vi "PID Online Autotuning (Relay Feedback).vi"(0 "setpoint":dbl(slide)=30.8641975308642 scale=0.0..100.0 scale format="%.1f", 1 "manipulated variable":dbl(slide)=30.8641975308642 scale=0.0..100.0 scale format="%.1f", 3 "autotuning parameters":T2={"type of controller"=1, "relay cycles"=3, "relay amplitude"=1.0, "control specifications"=2, "PV noise level"=0.1} {"PV noise level" format="%.2f"; "control specifications" items=["Fast", "Normal", "Slow"]; "relay amplitude" format="%.2f"; "type of controller" items=["P", "PI", "PID"]}, 5 "process variable":dbl(slide)=19.583333333333336 scale=0.0..100.0 scale format="%.1f", 9 "PID gains in":T1={"proportional gain (Kc)"=1.0, "integral time (Ti, min)"=0.01, "derivative time (Td, min)"=0.0} {"derivative time (Td, min)" format="%.3f"; "integral time (Ti, min)" format="%.3f"; "proportional gain (Kc)" format="%.3f"}, 11 "dt (s)":dbl=-1.0 format="%.3f", 12 "reinitialize? (F)":bool, 13 "autotune? (F)":bool) -> (4 "setpoint out":dbl(slide)=30.8641975308642 scale=0.0..100.0 scale format="%.1f", 6 "process variable out":dbl(slide)=19.583333333333336 scale=0.0..100.0 scale format="%.1f", 8 "tuning completed?":bool, 10 "PID gains out":T1={"proportional gain (Kc)"=1.0, "integral time (Ti, min)"=0.01, "derivative time (Td, min)"=0.0} {"derivative time (Td, min)" format="%.3f"; "integral time (Ti, min)" format="%.3f"; "proportional gain (Kc)" format="%.3f"}, 14 "tuned PID gains":T1={"proportional gain (Kc)"=1.0, "integral time (Ti, min)"=0.01, "derivative time (Td, min)"=0.0} {"derivative time (Td, min)" format="%.3f"; "integral time (Ti, min)" format="%.3f"; "proportional gain (Kc)" format="%.3f"})   [LabVIEW 2020, in "NI_PID_autopid.lvlib"]
doc: "Controls the parameters of a PID controller based on the autotuning technique of the polymorphic instance you select. You can use this VI in applications with other PID VIs, such as PID or PID Advanced, to construct and tune a PID controller. You must manually select the polymorphic instance to use."
uses:
  <vilib>/addons/control/pid/NI_PID_autopid.lvlib
  <vilib>/addons/control/pid/autopid.llb/PID autotuning parameters.ctl
  <vilib>/addons/control/pid/pid.llb/PID Structure Conversion (DBL).vi
  <vilib>/addons/control/pid/NI_PID_pid.lvlib
panel:
  in  "relay setpoint":bool
  in  "calculate parameters":bool
  # "Relay PID Auto Tune"
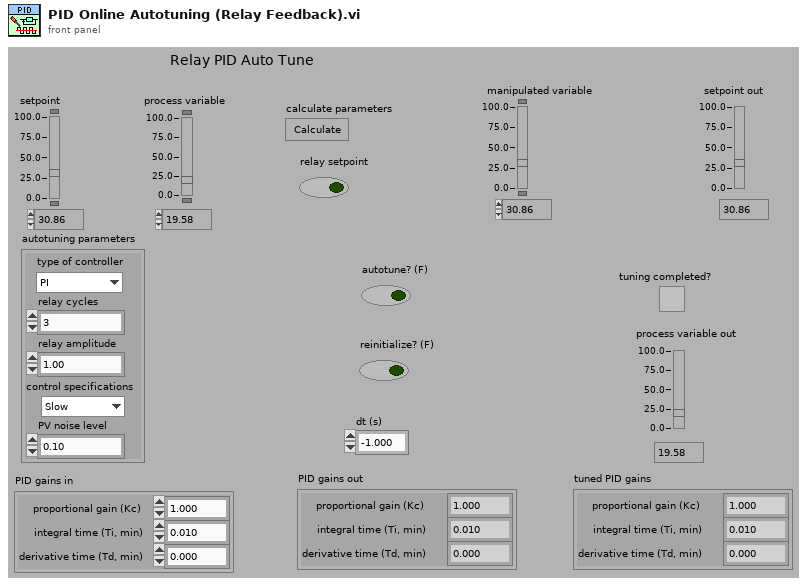
[diagram p1: front panel]
types:
  T1 = cluster{"proportional gain (Kc)":dbl, "integral time (Ti, min)":dbl, "derivative time (Td, min)":dbl}
  T2 = typedef "PID autotuning parameters.ctl" = cluster{"type of controller":u16, "relay cycles":i32, "relay amplitude":dbl, "control specifications":u16, "PV noise level":dbl}
  T3 = enum16{"Academic (Standard)", "Parallel", "Series"}
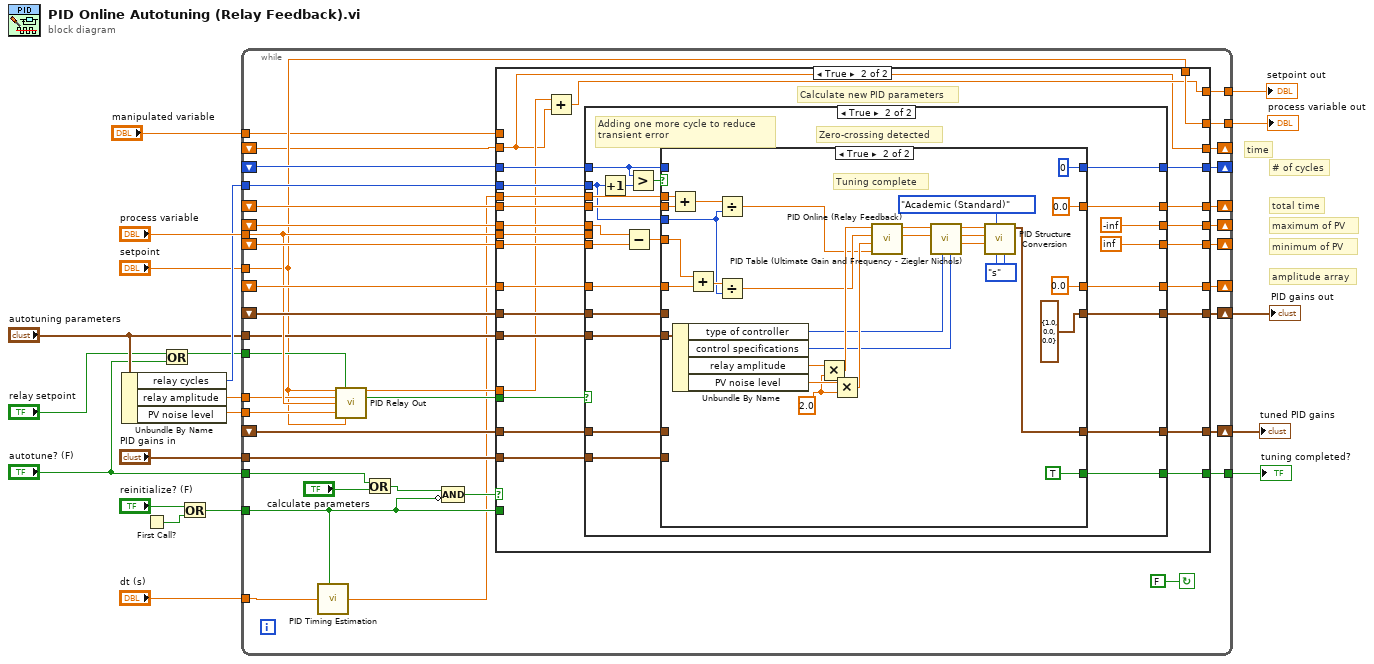
[diagram p0: block diagram]
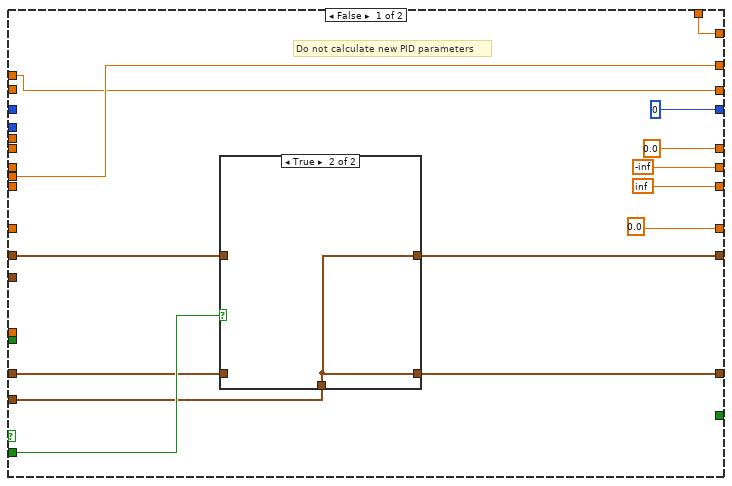
[diagram p2: hidden frame]
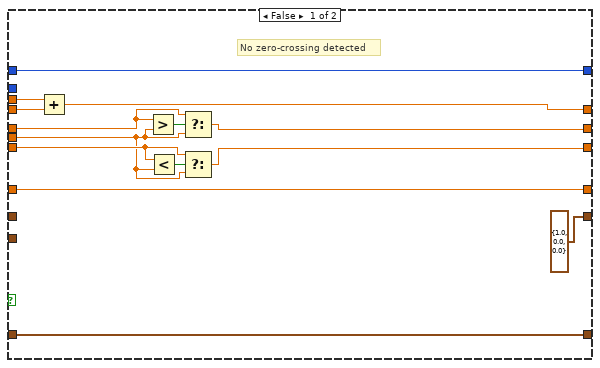
[diagram p4: hidden frame]
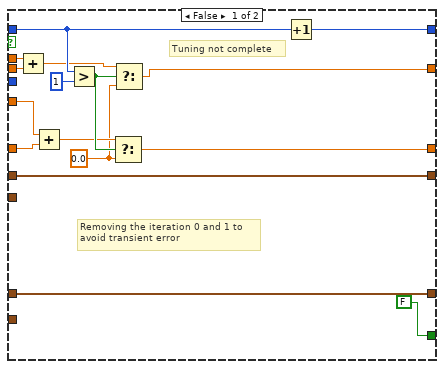
[diagram p5: hidden frame]
diagram:
  # "time"
  # "amplitude array"
  # "total time"
  # "minimum of PV"
  # "maximum of PV"
  # "# of cycles"
  n1 = Unbundle By Name("autotuning parameters") -> ("relay cycles"=w15:i32, "relay amplitude"=w11:dbl, "PV noise level"=w10:dbl)
  n2 = First Call?() -> (First Call?: T/F=w17:bool)
  n3 = Or(x="relay setpoint", y="autotune? (F)") -> (x .or. y?=w7:bool)
  n4 = Or(x="reinitialize? (F)", y=w17) -> (x .or. y?=w9:bool)
  n5 = while {
    shift-left: _ -> [w49]
    shift-right: [w48] -> _
    shift-left: _ -> [w50]
    shift-right: [w46] -> w20
    shift-left: _ -> [w53]
    shift-right: [w54] -> _
    shift-left: _ -> [w52]
    shift-right: [w55] -> _
    shift-left: _ -> [w56]
    shift-right: [w57] -> _
    shift-left: _ -> [w51]
    shift-right: [w58] -> _
    tunnel: w9 -> [w22]
    tunnel: "dt (s)" -> [w23]
    tunnel: "process variable" -> [w43]
    tunnel: w15 -> [w42]
    tunnel: w10 -> [w41]
    tunnel: w11 -> [w40]
    tunnel: "autotuning parameters" -> [w39]
    tunnel: "PID gains in" -> [w38]
    tunnel: "setpoint" -> [w32]
    tunnel: w7 -> [w37]
    tunnel: "autotune? (F)" -> [w34]
    tunnel: [w33] -> w5
    tunnel: [w30] -> w4
    tunnel: "manipulated variable" -> [w29]
    shift-right: [w28] -> _
    shift-left: _ -> [w27]
    tunnel: [w26] -> w2
    shift-right: [w25] -> w1
    shift-left: _ -> [w24]
    stop <- FALSE continue-if-true
    n6 = call <vilib>:"PID Timing Estimation.vi"("Initialize?"=w22, "dt (s) in"=w23) -> ("dt (s) out"=w21:dbl)  [unwired: 7 in]
    n7 = call <vilib>:"PID Relay Out.vi"("Setpoint Reference"=w32, "Relay Setpoint"=w37, "Relay Amplitude"=w40, "Process Variable"=w43, "Noise Disturbance"=w41, "Process Variable Reference"=w32) -> ("relay output"=w31:dbl, "Zero Crossing"=w36:bool)  [unwired: 2 in, 6 out]
    n8 = Or(x=w34, y="calculate parameters") -> (x .or. y?=w35:bool)
    n9 = Compound Arithmetic op=AND(w35, invert w22) -> (w44:bool)
    n10 = case shown="True" w44 {
      tunnel: w51 -> [_ w89]
      tunnel: [0 w90] -> w58
      tunnel: [-inf w91] -> w57
      tunnel: w56 -> [_ w100]
      tunnel: w52 -> [_ w99]
      tunnel: [0.0 w93] -> w55
      tunnel: [inf w92] -> w54
      tunnel: w53 -> [_ w94]
      tunnel: w42 -> [_ w98]
      tunnel: [w61 w95] -> w46
      tunnel: w50 -> [w60 w83]
      tunnel: w36 -> [_ w97]
      tunnel: w21 -> [_ w96]
      tunnel: w49 -> [_ w88]
      tunnel: [0.0 ("f") w87] -> w48
      tunnel: w39 -> [_ w86]
      tunnel: w38 -> [w67 w85]
      tunnel: w22 -> [w68 _]
      tunnel: w43 -> [w65 w84]
      tunnel: [w65 w82] -> w33
      tunnel: w32 -> [w64 w82]
      tunnel: w31 -> [_ w81]
      tunnel: [w64 w80] -> w30
      tunnel: w29 -> [w63 _]
      tunnel: [w63 w79] -> w28
      tunnel: w27 -> [_ w79]
      tunnel: [_ w78] -> w26
      tunnel: [w59 w77] -> w25
      tunnel: w24 -> [w62 w76]
      frame False {
        # "Do not calculate new PID parameters"
        n11 = case shown="True" w68 {
          tunnel: [w73 w75] -> w61
          tunnel: w62 -> [w74 _]
          tunnel: w67 -> [w73 w75]
          tunnel: w60 -> [_ _]
          tunnel: [w74 w75] -> w59
          frame False {
          }
          frame True {
          }
        }
      }
      frame True {
        # "Calculate new PID parameters"
        n12 = Add(x=w81, y=w79) -> (x+y=w80:dbl)
        n13 = case shown="True" w97 {
          tunnel: w89 -> [w114 w124]
          tunnel: [w114 w126] -> w90
          tunnel: [w113 -inf] -> w91
          tunnel: w100 -> [w112 w136]
          tunnel: w99 -> [w111 w134]
          tunnel: [w111 w132] -> w93
          tunnel: [w108 inf] -> w92
          tunnel: w94 -> [w109 w135]
          tunnel: w98 -> [_ w121]
          tunnel: w83 -> [_ w131]
          tunnel: w96 -> [w105 w130]
          tunnel: [cluster{"Kc":dbl, "Ti":dbl, "Td":dbl} {"Kc"=1.0, "Ti"=0.0, "Td"=0.0} ("tuned PID parameters") w129] -> w95
          tunnel: w88 -> [w106 w123]
          tunnel: [w104 w122] -> w87
          tunnel: w86 -> [_ w120]
          tunnel: w85 -> [_ w119]
          tunnel: w84 -> [w102 _]
          tunnel: [_ w117] -> w78
          tunnel: [w101 w116] -> w77
          tunnel: w76 -> [w101 w115]
          frame False {
            # "No zero-crossing detected"
            n14 = Add(x=w105, y=w106) -> (x+y=w104:dbl)
            n15 = Greater?(x=w112, y=w102) -> (0:w107:bool)
            n16 = Less?(x=w109, y=w102) -> (x < y?=w110:bool)
            n17 = Select(t=w112, s=w107, f=w102) -> (s? t:f=w113:dbl)
            n18 = Select(t=w109, s=w110, f=w102) -> (s? t:f=w108:dbl)
          }
          frame True {
            # "Adding one more cycle to reduce\ntransient error"
            # "Zero-crossing detected"
            n19 = Increment(x=w121) -> (x+1=w118:i32)
            n20 = Subtract(x=w136, y=w135) -> (x-y=w133:dbl)
            n21 = Greater?(x=w124, y=w118) -> (0:w125:bool)
            n22 = case shown="True" w125 {
              tunnel: w134 -> [w146 w174]
              tunnel: w133 -> [w147 w175]
              tunnel: [w141 0.0] -> w132
              tunnel: [w138 0] -> w126
              tunnel: w124 -> [w145 _]
              tunnel: [FALSE TRUE] -> w117
              tunnel: [w152 cluster{"Kc":dbl, "Ti":dbl, "Td":dbl} {"Kc"=1.0, "Ti"=0.0, "Td"=0.0} ("tuned PID parameters")] -> w129
              tunnel: w131 -> [w152 _]
              tunnel: w130 -> [w151 w178]
              tunnel: w123 -> [w150 w179]
              tunnel: [w149 0.0 ("f")] -> w122
              tunnel: w121 -> [_ w172]
              tunnel: w120 -> [_ w170]
              tunnel: w119 -> [_ _]
              tunnel: [w137 w156] -> w116
              tunnel: w115 -> [w137 _]
              frame False {
                w140 = 0.0 ("f")
                # "Removing the iteration 0 and 1 to \navoid transient error"
                # "Tuning not complete"
                n23 = Add(x=w151, y=w150) -> (x+y=w139:dbl)
                n24 = Add(x=w147, y=w146) -> (x+y=w142:dbl)
                n25 = Greater?(x=w145, y=1) -> (0:w143:bool)
                n26 = Select(t=w142, s=w143, f=w140) -> (s? t:f=w141:dbl)
                n27 = Select(t=w139, s=w143, f=w140) -> (s? t:f=w149:dbl)
                n28 = Increment(x=w145) -> (x+1=w138:i32)
              }
              frame True {
                w154 = enum16{"min", "s"}."s" ("integral unit")
                w153 = 2.0 ("y")
                # "Tuning complete"
                n29 = Add(x=w178, y=w179) -> (x+y=w177:dbl)
                n30 = Unbundle By Name(w170) -> ("type of controller"=w162:u16, "control specifications"=w161:u16, "relay amplitude"=w169:dbl, "PV noise level"=w168:dbl)
                n31 = Add(x=w175, y=w174) -> (x+y=w173:dbl)
                n32 = Divide(x=w177, y=w172) -> (x/y=w160:dbl)
                n33 = Divide(x=w173, y=w172) -> (x/y=w165:dbl)
                n34 = Multiply(x=w169, y=w153) -> (x*y=w166:dbl)
                n35 = Multiply(x=w168, y=w153) -> (x*y=w167:dbl)
                n36 = call <vilib>:"PID Online (Relay Feedback).vi"("Period"=w160, "Noise level (e)"=w167, "Output amplitude (a)"=w165, "Relay Input amplitude (d)"=w166) -> ("Ultimate Period (Tu)"=w163:dbl, "Ultimate Gain (Ku)"=w164:dbl)  [unwired: 5 in, 1 out]
                n37 = call <vilib>:"PID Table (Ultimate Gain and Frequency - Ziegler Nichols).vi"("Control Design"=w161, "Type of Controller"=w162, "Ultimate Period (Tu)"=w163, "Ultimate Gain (Ku)"=w164) -> ("Derivative Time (Td)"=w157:dbl, "Integral Time (Ti)"=w158:dbl, "Proportional Gain (Kp)"=w159:dbl)  [unwired: 5 in]
                n38 = call-poly <vilib>:"PID Structure Conversion.vi"("derivative unit"=w154, "integral unit"=w154, "PID structure"=T3."Academic (Standard)", "derivative"=w157, "integral"=w158, "proportional"=w159) -> ("PID gains"=w156:T1)  [unwired: 5 in]
              }
            }
          }
        }
      }
    }
  }
  "PID gains out" <- w20
  "process variable out" <- w5
  "setpoint out" <- w4
  "tuning completed?" <- w2
  "tuned PID gains" <- w1
